vi "Mapping Simulated Spectrum v10.1.0.vi"() -> (0 "Simulated Spectrum":cluster{i32[], dbl[]}[](array[cluster]))   [LabVIEW 2010]
panel:
  out "Y (2D)":dbl[](array[numeric])
  out "X (1D)":i32[](array[numeric])
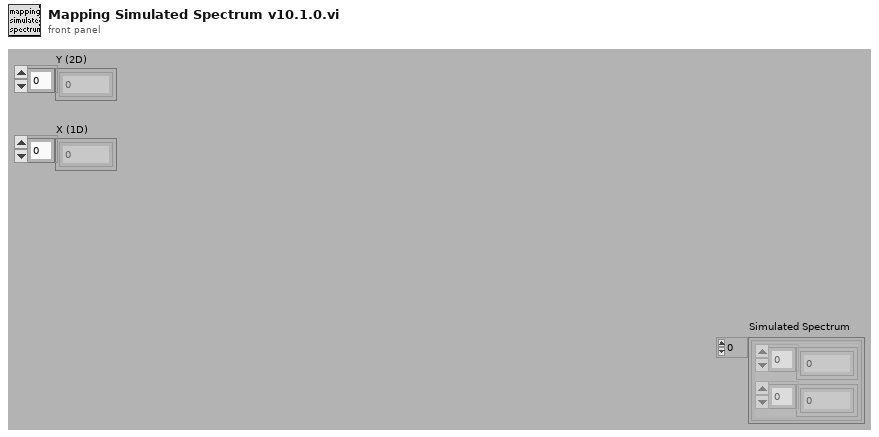
[diagram p1: front panel]
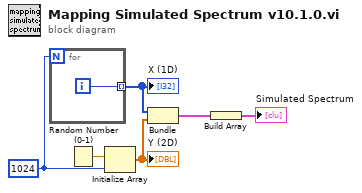
[diagram p0: block diagram]
diagram:
  w6 = 1024 ("Dimension")
  n1 = for {
    N: w6 -> [_]
    tunnel: [w7] -> w4 mode=indexing
    i -> [w7]
  }
  "X (1D)" <- w4
  n2 = Random Number (0-1)() -> (number: 0 to 1=w5:dbl)
  n3 = Initialize Array(w5, w6) -> (w3:dbl[])
  "Y (2D)" <- w3
  n4 = Bundle(w4, w3) -> (w2:cluster{i32[], dbl[]})  [unwired: 1 in]
  n5 = Build Array(w2) -> (→"Simulated Spectrum":cluster{i32[], dbl[]}[])
